vi "OSC_Calc_Digital.vi"(8 "Flow":dbl, 9 "Lambda 2 Array":dbl[](array[numeric]), 10 "Lambda 1 Array":dbl[](array[numeric]), 11 "MFC":dbl) -> (0 "OSC MFC":dbl, 1 "OSC-Meas Flow":dbl, 2 "OSC- Calc Flow":dbl, 3 "Calculated Flow":dbl, 4 "Time":dbl)   [LabVIEW 2014]
uses:
  <vilib>/Analysis/baseanly.llb/Mean (DBL).vi
  <vilib>/Analysis/NI_AALPro.lvlib
  <vilib>/Analysis/NI_AALBase.lvlib
panel:
  out "L1 TP 2":i32
  out "Value 2":dbl
  out "L2 TP 2":i32
  out "Value":dbl
  out "mean":dbl format="%0.2f"
  out "mean 2":dbl format="%0.2f"
  out "mean 3":dbl format="%0.2f"
  out "L1 Gradient":dbl[](graph)
  out "L1 Gradient dy/dx":dbl[](graph)
  out "L1 Data":dbl[](graph)
  out "L1 Max Grad":dbl
  out "L1 TP":i32
  out "L2 Gradient":dbl[](graph)
  out "L2 Gradient dy/dx":dbl[](graph)
  out "L2 Data":dbl[](graph)
  out "L2 Max Grad":dbl
  out "L2 TP":i32
  # "OSC Calculation"
  # "Inputs"
  # "Outputs"
  # "Indicators"
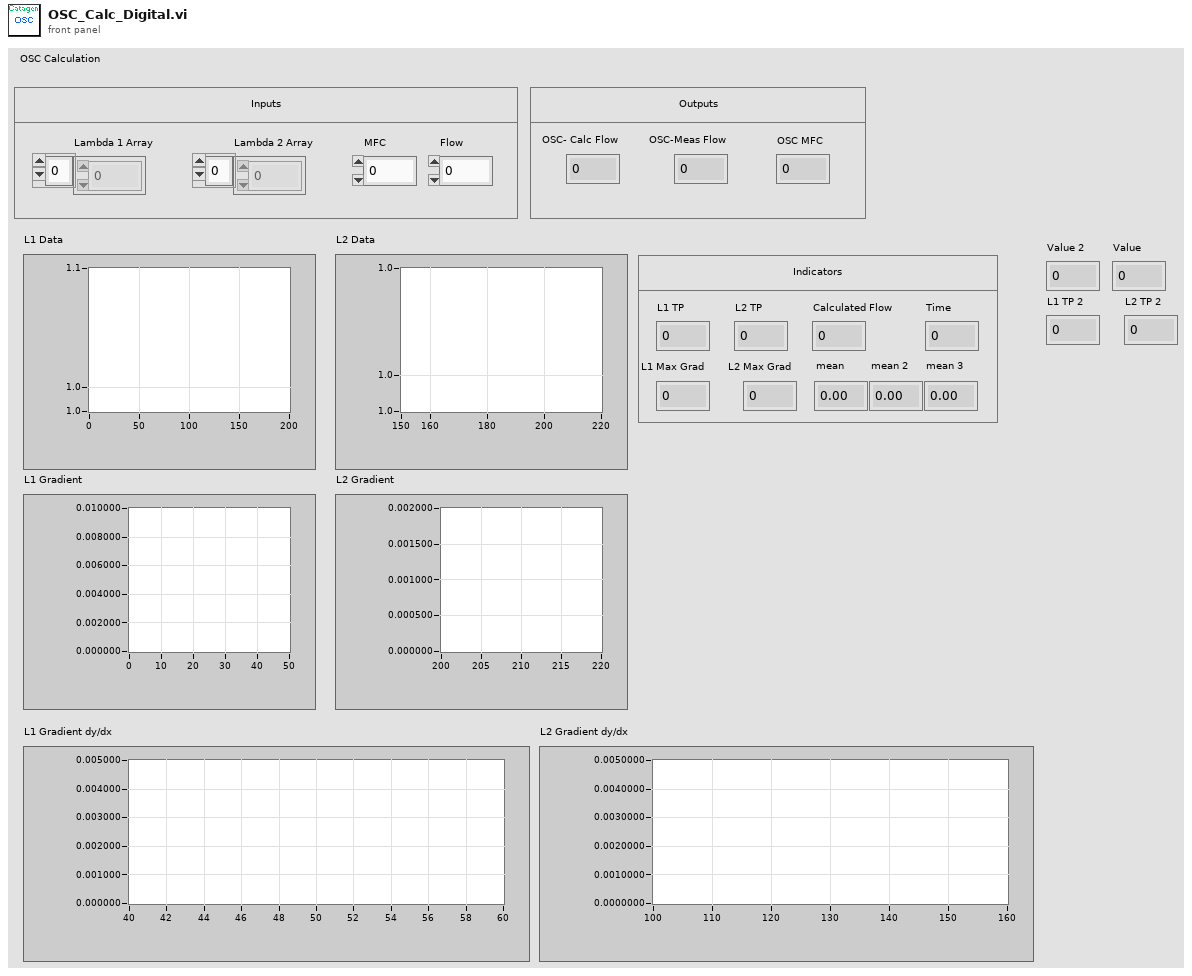
[diagram p1: front panel]
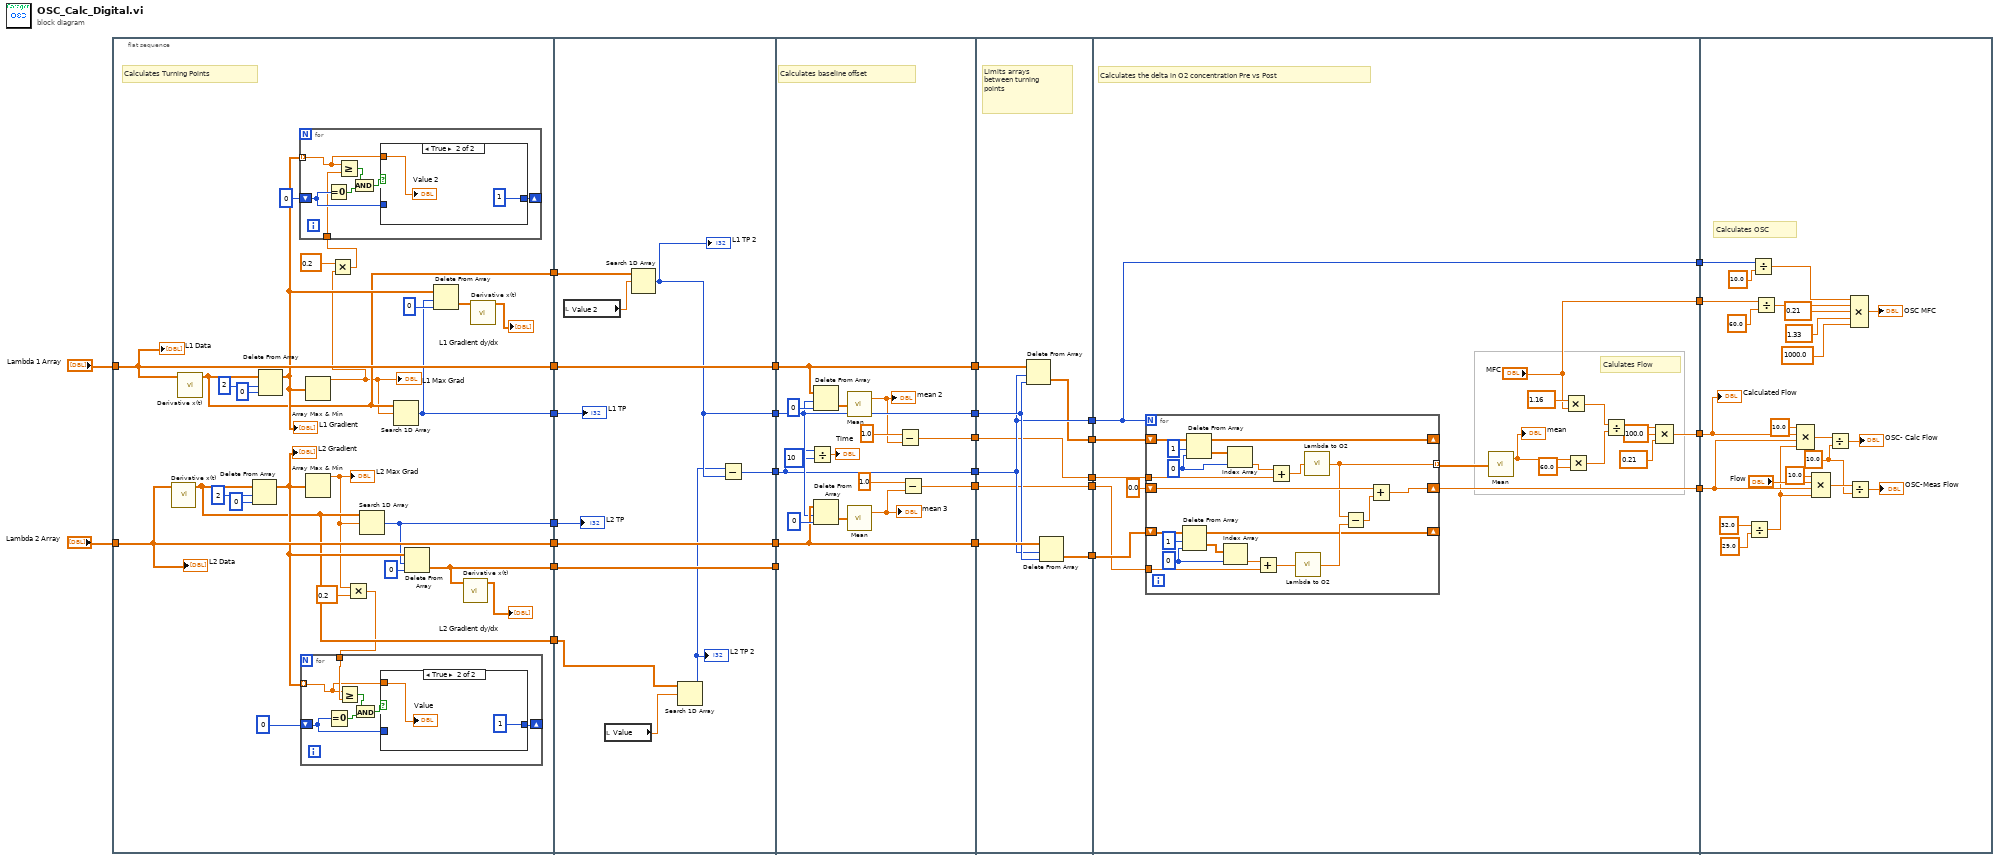
[diagram p0: block diagram]
diagram:
  n1 = flat-sequence {
    tunnel: [w49] -> w12
    tunnel: [w51] -> w10
    tunnel: "Lambda 1 Array" -> [w51]
    tunnel: "Lambda 2 Array" -> [w49]
    tunnel: [w48] -> w6
    tunnel: [w41] -> w4
    tunnel: [w39] -> w3
    tunnel: [w32] -> w2
    tunnel: [w31] -> w1
    tunnel: w12 -> [w87]
    tunnel: [w87] -> w11
    tunnel: w10 -> [w86]
    tunnel: [w86] -> w9
    tunnel: [w83] -> w8
    tunnel: [w77] -> w7
    tunnel: w6 -> [w85]
    tunnel: [w85] -> w5
    tunnel: w4 -> [w78]
    tunnel: w3 -> [w80]
    tunnel: w2 -> [w84]
    tunnel: w1 -> [w82]
    tunnel: w11 -> [w98]
    tunnel: [w98] -> w29
    tunnel: w9 -> [w103]
    tunnel: [w103] -> w28
    tunnel: w8 -> [w90]
    tunnel: [w90] -> w27
    tunnel: w7 -> [w97]
    tunnel: [w97] -> w26
    tunnel: [w95] -> w25
    tunnel: [w91] -> w16
    tunnel: w5 -> [_]
    tunnel: w29 -> [w110]
    tunnel: w28 -> [w111]
    tunnel: w27 -> [w108]
    tunnel: w26 -> [w109]
    tunnel: [w108] -> w24
    tunnel: [w107] -> w23
    tunnel: [w106] -> w22
    tunnel: w25 -> [w105]
    tunnel: [w105] -> w21
    tunnel: w16 -> [w104]
    tunnel: [w104] -> w15
    tunnel: w24 -> [w113]
    tunnel: w23 -> [w128]
    tunnel: w22 -> [w129]
    tunnel: [w126] -> w20
    tunnel: [w116] -> w19
    tunnel: w21 -> [w115]
    tunnel: w15 -> [w114]
    tunnel: ["MFC"] -> w14
    tunnel: [w113] -> w13
    tunnel: w20 -> [w168]
    tunnel: w19 -> [w172]
    tunnel: w14 -> [w158]
    tunnel: w13 -> [w154]
    frame #0 {
      # "Calculates Turning Points"
      n2 = call <vilib>:"Derivative x(t).vi"("X"=w49) -> ("dX/dt"=w41:dbl[])  [unwired: 9 in, 1 out]
      n3 = call <vilib>:"Derivative x(t).vi"("X"=w51) -> ("dX/dt"=w39:dbl[])  [unwired: 9 in, 1 out]
      n4 = Delete From Array(array=w41, length=2, index=0) -> (array with subset deleted=w43:dbl[])  [unwired: 1 out]
      "L2 Gradient" <- w43
      n5 = Delete From Array(array=w39, length=2, index=0) -> (array with subset deleted=w40:dbl[])  [unwired: 1 out]
      "L1 Gradient" <- w40
      n6 = Array Max & Min(array=w40) -> (max value=w34:dbl)  [unwired: 3 out]
      "L1 Max Grad" <- w34
      n7 = Array Max & Min(array=w43) -> (max value=w38:dbl)  [unwired: 3 out]
      "L2 Max Grad" <- w38
      n8 = Multiply(x=0.2, y=w34) -> (x*y=w35:dbl)
      n9 = for {
        tunnel: w40 -> [w58] mode=indexing
        shift-right: [w60] -> _
        shift-left: 0 ("index") -> [w57]
        tunnel: w35 -> [w56]
        n10 = Equal To 0?(x=w57) -> (x = 0?=w59:bool)
        n11 = Greater Or Equal?(x=w58, y=w56) -> (x >= y?=w61:bool)
        n12 = And(x=w61, y=w59) -> (x .and. y?=w62:bool)
        n13 = case shown="True" w62 {
          tunnel: [w63 1 ("index")] -> w60
          tunnel: w58 -> [_ w64]
          tunnel: w57 -> [w63 _]
          frame False {
          }
          frame True {
            "Value 2" <- w64
          }
        }
      }
      n14 = Multiply(x=w38, y=0.2) -> (x*y=w37:dbl)
      n15 = for {
        tunnel: w37 -> [w72]
        tunnel: w43 -> [w67] mode=indexing
        shift-right: [w69] -> _
        shift-left: 0 ("index") -> [w66]
        n16 = Equal To 0?(x=w66) -> (x = 0?=w68:bool)
        n17 = Greater Or Equal?(x=w67, y=w72) -> (x >= y?=w70:bool)
        n18 = And(x=w70, y=w68) -> (x .and. y?=w71:bool)
        n19 = case shown="True" w71 {
          tunnel: [w73 1 ("index")] -> w69
          tunnel: w67 -> [_ w74]
          tunnel: w66 -> [w73 _]
          frame False {
          }
          frame True {
            "Value" <- w74
          }
        }
      }
      n20 = Search 1D Array(1D array=w41, element=w38) -> (index of element=w31:i32)  [unwired: 1 in]
      n21 = Search 1D Array(1D array=w39, element=w34) -> (index of element=w32:i32)  [unwired: 1 in]
      n22 = Delete From Array(array=w43, length=w31, index=0) -> (deleted portion=w48:dbl[])  [unwired: 1 out]
      n23 = Delete From Array(array=w40, length=w32, index=0) -> (deleted portion=w46:dbl[])  [unwired: 1 out]
      n24 = call <vilib>:"Derivative x(t).vi"("X"=w48) -> ("dX/dt"=→"L2 Gradient dy/dx":dbl[])  [unwired: 9 in, 1 out]
      n25 = call <vilib>:"Derivative x(t).vi"("X"=w46) -> ("dX/dt"=→"L1 Gradient dy/dx":dbl[])  [unwired: 9 in, 1 out]
      "L1 Data" <- w51
      "L2 Data" <- w49
    }
    frame #1 {
      n26 = local read "Value 2"() -> (w81:dbl)
      n27 = local read "Value"() -> (w79:dbl)
      n28 = Search 1D Array(1D array=w80, element=w81) -> (index of element=w77:i32)  [unwired: 1 in]
      "L1 TP 2" <- w77
      n29 = Search 1D Array(1D array=w78, element=w79) -> (index of element=w76:i32)  [unwired: 1 in]
      "L2 TP 2" <- w76
      n30 = Subtract(x=w76, y=w77) -> (x-y=w83:i32)
      "L1 TP" <- w84
      "L2 TP" <- w82
    }
    frame #2 {
      # "Calculates baseline offset"
      n31 = Divide(x=w90, y=10) -> (x/y=→"Time":dbl)
      n32 = Delete From Array(array=w103, length=w97, index=0) -> (deleted portion=w101:dbl[])  [unwired: 1 out]
      n33 = Delete From Array(array=w98, length=w97, index=0) -> (deleted portion=w100:dbl[])  [unwired: 1 out]
      n34 = call-poly <vilib>:"Mean.vi"("X"=w101) -> ("mean"=w93:dbl)  [unwired: 1 out]
      "mean 2" <- w93
      n35 = call-poly <vilib>:"Mean.vi"("X"=w100) -> ("mean"=w96:dbl)  [unwired: 1 out]
      "mean 3" <- w96
      n36 = Subtract(x=1.0, y=w93) -> (x-y=w91:dbl)
      n37 = Subtract(x=1.0, y=w96) -> (x-y=w95:dbl)
    }
    frame #3 {
      # "Limits arrays\nbetween turning\npoints"
      n38 = Delete From Array(array=w111, length=w108, index=w109) -> (deleted portion=w106:dbl[])  [unwired: 1 out]
      n39 = Delete From Array(array=w110, length=w108, index=w109) -> (deleted portion=w107:dbl[])  [unwired: 1 out]
    }
    frame #4 {
      # "Calculates the delta in O2 concentration Pre vs Post"
      # "Calulates Flow"
      n40 = for {
        N: w113 -> [_]
        shift-right: [w137] -> _
        shift-left: w129 -> [w150]
        shift-right: [w136] -> _
        shift-left: w128 -> [w143]
        shift-right: [w141] -> w126
        shift-left: 0.0 ("element") -> [w142]
        tunnel: [w138] -> w125 mode=indexing
        tunnel: w115 -> [w134]
        tunnel: w114 -> [w131]
        w146 = 0 ("index")
        w147 = 0 ("index")
        n41 = Delete From Array(array=w143, length=1, index=w146) -> (deleted portion=w145:dbl[], array with subset deleted=w136:dbl[])
        n42 = Delete From Array(array=w150, length=1, index=w147) -> (deleted portion=w148:dbl[], array with subset deleted=w137:dbl[])
        n43 = Index Array(array=w145, index=w146) -> (element=w135:dbl)
        n44 = Index Array(array=w148, index=w147) -> (element=w132:dbl)
        n45 = Add(x=w135, y=w134) -> (x+y=w133:dbl)
        n46 = Add(x=w132, y=w131) -> (x+y=w130:dbl)
        n47 = call "Lambda to O2.vi"("Lambda"=w133) -> ("O2 %"=w139:sgl)
        n48 = call "Lambda to O2.vi"("Lambda"=w130) -> ("O2 %"=w138:sgl)
        n49 = Subtract(x=w138, y=w139) -> (x-y=w140:sgl)
        n50 = Add(x=w142, y=w140) -> (x+y=w141:dbl)
      }
      n51 = call-poly <vilib>:"Mean.vi"("X"=w125) -> ("mean"=w123:dbl)  [unwired: 1 out]
      "mean" <- w123
      n52 = Multiply(x=1.16, y="MFC") -> (x*y=w121:dbl)
      n53 = Multiply(x=w123, y=60.0) -> (x*y=w120:dbl)
      n54 = Divide(x=w121, y=w120) -> (x/y=w119:dbl)
      n55 = Compound Arithmetic op=MULTIPLY(w119, 100.0 ("value"), 0.21 ("value")) -> (w116:dbl)
    }
    frame #5 {
      w161 = 10.0 ("y")
      # "Calculates OSC"
      n56 = Divide(x=32.0, y=29.0) -> (x/y=w166:dbl)
      n57 = Divide(x=w154, y=10.0) -> (x/y=w152:dbl)
      n58 = Divide(x=w158, y=60.0) -> (x/y=w159:dbl)
      n59 = Compound Arithmetic op=MULTIPLY(10.0 ("value"), w172, w168, w166) -> (w162:dbl)
      n60 = Compound Arithmetic op=MULTIPLY(10.0 ("value"), "Flow", w168, w166) -> (w163:dbl)
      n61 = Divide(x=w162, y=w161) -> (x/y=→"OSC- Calc Flow":dbl)
      n62 = Divide(x=w163, y=w161) -> (x/y=→"OSC-Meas Flow":dbl)
      n63 = Compound Arithmetic op=MULTIPLY(w152, w159, 0.21 ("value"), 1.33 ("value"), 1000.0 ("value")) -> (→"OSC MFC":dbl)
      "Calculated Flow" <- w172
    }
  }
